vi "Determine Elf Move.vi"(5 "Grove":T3[][](array[typedef]), 7 "Eff ID":i32, 8 "Proposed Direction List":T4[](array[typedef]), 10 "Point":T2, 11 "Move Map":T1) -> (3 "Move Map Out":T1)   [LabVIEW 2020]
uses:
  Cluster _Point Location.ctl
  ENUM_Location Direction.ctl
  RB ENUM_Spot ID.ctl
  MAP_Poroposed Moves.ctl
  <vilib>/Utility/miscctls.llb/LVMapReplaceAction.ctl
panel:
  out "New Move":bool
  out "Elf Found Out":bool
  out "Direction":T4
  out "New Position":T2
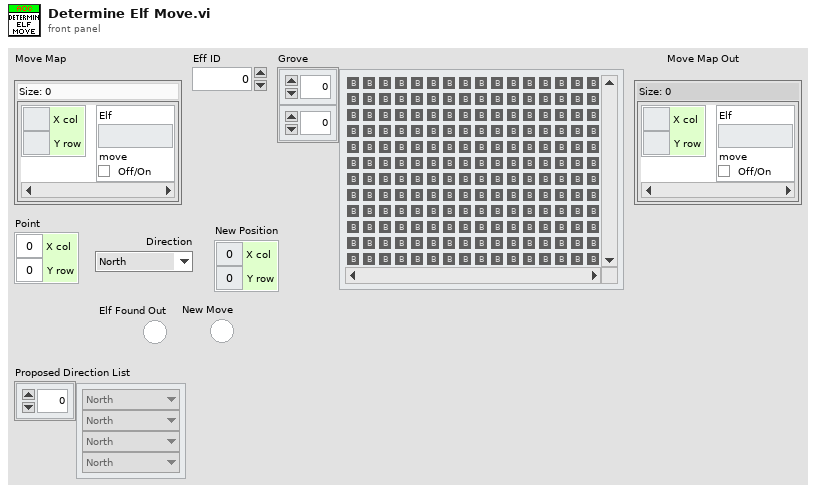
[diagram p1: front panel]
types:
  T1 = typedef "MAP_Poroposed Moves.ctl" = map{T2, cluster{"Elf":i32, "move":bool}}
  T2 = typedef "Cluster _Point Location.ctl" = cluster{"X col":i32, "Y row":i32}
  T3 = typedef "RB ENUM_Spot ID.ctl" = enum32{"Blank", "ELF", "Proposed"}
  T4 = typedef "ENUM_Location Direction.ctl" = enum16{"North", "North-East", "East", "South-East", "South", "South-West", "West", "North-West", "Center"}
  T5 = typedef "LVMapReplaceAction.ctl" = enum32{"Modify Entry only if found", "Add or Modify Entry", "Delete Entry"}
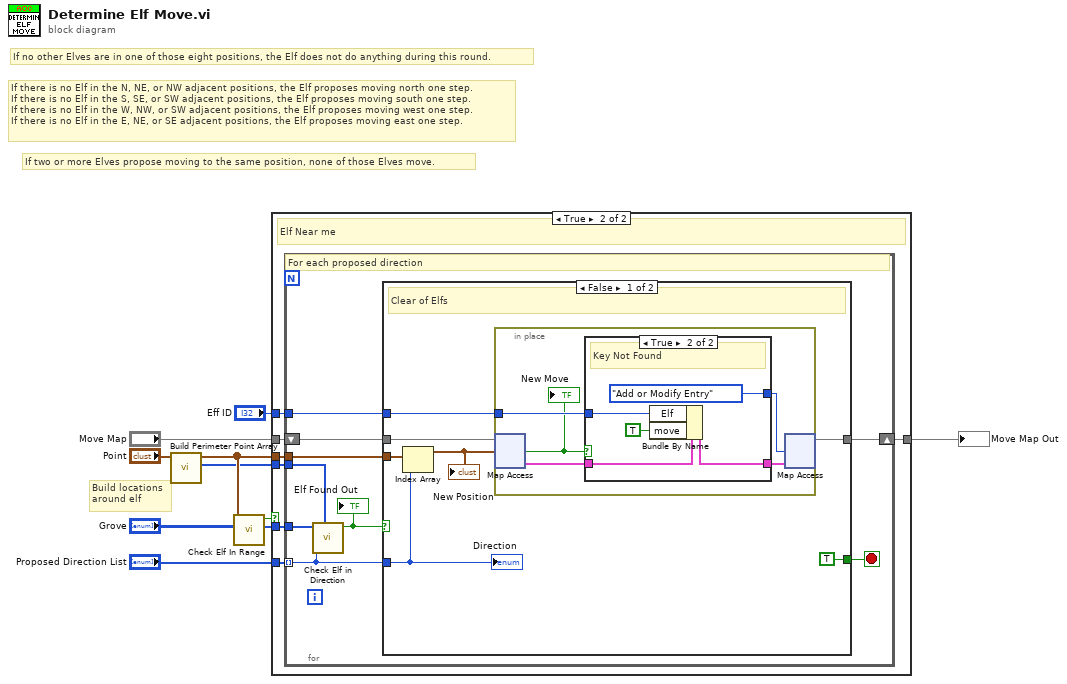
[diagram p0: block diagram]
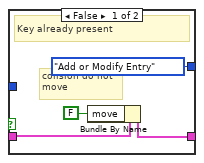
[diagram p3: hidden frame]
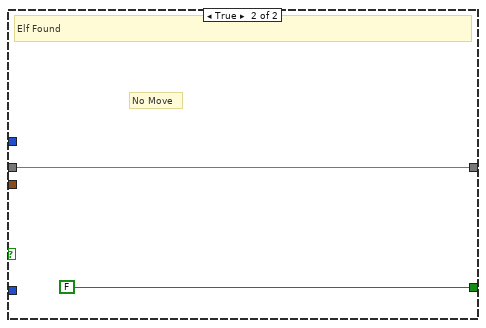
[diagram p4: hidden frame]
diagram:
  # "Build locations\naround elf"
  # "If two or more Elves propose moving to the same position, none of those Elves move."
  # "If there is no Elf in the N, NE, or NW adjacent positions, the Elf proposes moving north one step.\nIf there is no Elf in the S, SE, or SW adjacent positions, the Elf proposes moving south one step.\nIf there is no Elf in the W, NW, or SW adjacent positions, the Elf proposes moving west one step.\nIf there is no Elf in the E, NE, or SE adjacent positions, the Elf proposes moving east one step."
  # "If no other Elves are in one of those eight positions, the Elf does not do anything during this round."
  n1 = call "Build Perimeter Point Array.vi"("Start Point"="Point") -> ("List No Center Out"=w1:T4[], "No Center Out"=w8:T2[])  [unwired: 7 in, 2 out]
  n2 = call "Check Elf In Range.vi"("Grove"="Grove", "Elf Position"=w8) -> ("Elf Present array"=w4:T3[], "Elf  in Range"=w2:bool)  [unwired: 8 in]
  n3 = case shown="True" w2 {
    tunnel: "Move Map" -> [w11 w16]
    tunnel: w4 -> [_ w18]
    tunnel: [w11 w15] -> w5
    tunnel: w8 -> [_ w14]
    tunnel: "Proposed Direction List" -> [_ w17]
    tunnel: "Eff ID" -> [_ w13]
    tunnel: w1 -> [_ w12]
    frame False {
      # "No Move"
      # "No Elfs Near me"
    }
    frame True {
      # "Elf Near me"
      n4 = for {
        tunnel: w18 -> [w27]
        tunnel: w17 -> [w20] mode=indexing
        shift-right: [w23] -> w15
        shift-left: w16 -> [w24]
        tunnel: w14 -> [w22]
        tunnel: w13 -> [w21]
        tunnel: w12 -> [w19]
        stop <- w25 stop-if-true
        # "For each proposed direction"
        n5 = call "Check Elf in Direction.vi"("List No Center Out"=w19, "Direction"=w20, "Elf Present Array"=w27) -> ("Elf Found Out"=w26:bool)  [unwired: 7 in, 1 out]
        "Elf Found Out" <- w26
        n6 = case shown="False" w26 {
          tunnel: [TRUE FALSE] -> w25
          tunnel: w20 -> [w33 _]
          tunnel: w24 -> [w31 w50]
          tunnel: [w30 w50] -> w23
          tunnel: w22 -> [w34 _]
          tunnel: w21 -> [w29 _]
          frame False {
            # "Clear of Elfs"
            n7 = Index Array(array=w34, index=w33) -> (element=w28:T2)
            "New Position" <- w28
            n8 = in-place {
              in-place-border: w29 -> [w39]
              n9 = in-place-map #1(w31, w28) -> (w37:cluster{"Elf":i32, "move":bool}, w38:bool)  [unwired: 1 in]
              "New Move" <- w38
              n10 = case shown="True" w38 {
                tunnel: w39 -> [_ w45]
                tunnel: w37 -> [w43 w47]
                tunnel: [w40 w44] -> w36
                tunnel: [LVMapReplaceAction."Add or Modify Entry" ("action") LVMapReplaceAction."Add or Modify Entry" ("action")] -> w35
                frame False {
                  # "colision do not\nmove"
                  # "Key already present"
                  n11 = Bundle By Name(cluster=w43, "move"=FALSE) -> (w40:cluster{"Elf":i32, "move":bool})
                }
                frame True {
                  # "Key Not Found"
                  n12 = Bundle By Name(cluster=w47, "Elf"=w45, "move"=TRUE) -> (w44:cluster{"Elf":i32, "move":bool})
                }
              }
              n13 = in-place-map #1(w36, w35) -> (w30:T1)  [unwired: 2 out]
            }
            "Direction" <- w33
          }
          frame True {
            # "No Move"
            # "Elf Found"
          }
        }
      }
    }
  }
  "Move Map Out" <- w5
